vi "IIR_test.vi"() -> ()   [LabVIEW 2017]
uses:
  <vilib>/Analysis/4window.llb/windowTd.ctl
  <vilib>/Utility/file.llb/Read Delimited Spreadsheet (DBL).vi
  <vilib>/Analysis/3filter.llb/IIR Filter (DBL).vi
  <vilib>/measure/maspectr.llb/FFT Spectrum (Mag-Phase) for 1 Chan.vi
  <vilib>/measure/NI_MAPro.lvlib
  <vilib>/Analysis/NI_AALPro.lvlib
  <vilib>/Analysis/NI_AALBase.lvlib
  <vilib>/measure/NI_MABase.lvlib
panel:
  out "Phase 3":cluster{"f0":dbl, "df":dbl, "magnitude":dbl[]}(graph)
  out "Magnitude 3":cluster{"f0":dbl, "df":dbl, "magnitude":dbl[]}(graph)
  out "Waveform Graph 3":waveform(dbl)(graph)
  out "error":i32
  out "Phase 2":cluster{"f0":dbl, "df":dbl, "magnitude":dbl[]}(graph)
  out "Magnitude 2":cluster{"f0":dbl, "df":dbl, "magnitude":dbl[]}(graph)
  out "Waveform Graph 2":waveform(dbl)(graph)
  out "Phase":cluster{"f0":dbl, "df":dbl, "magnitude":dbl[]}(graph)
  out "Magnitude":cluster{"f0":dbl, "df":dbl, "magnitude":dbl[]}(graph)
  out "Waveform Graph":waveform(dbl)(graph)
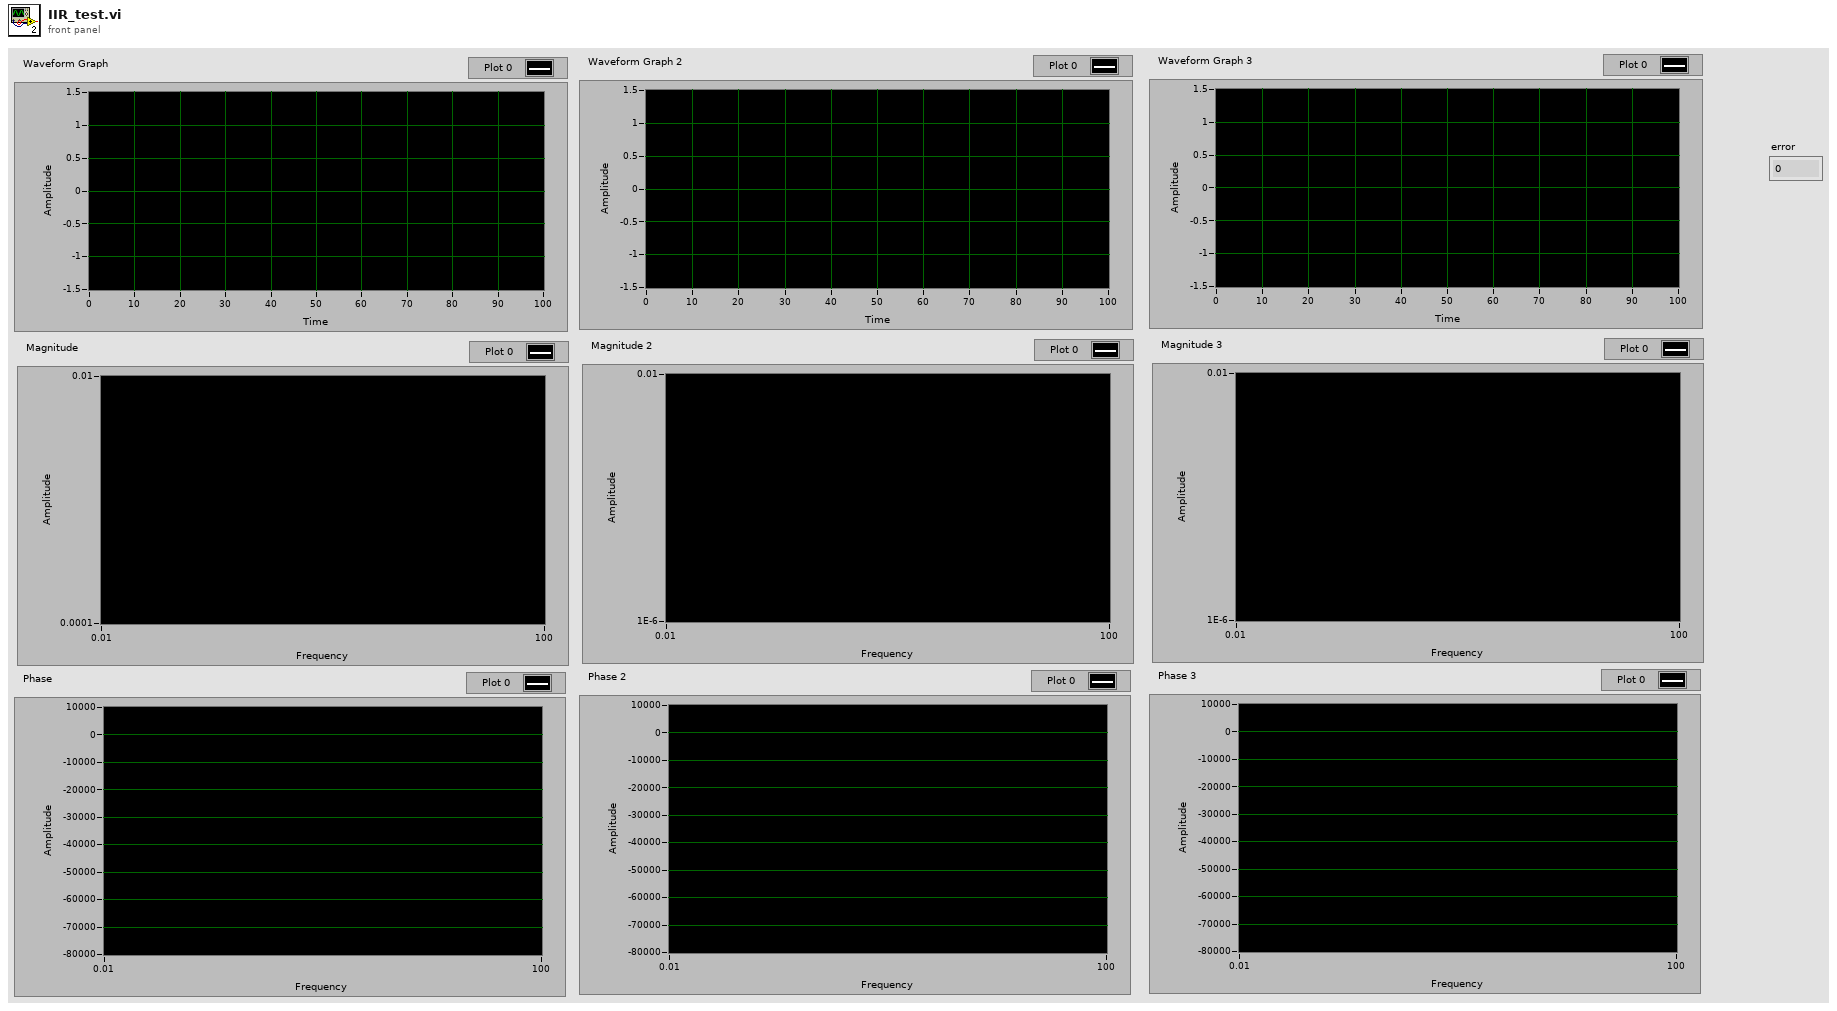
[diagram p1: front panel]
types:
  T1 = typedef "NI_AALPro.lvlib/windowTd.ctl" = u32
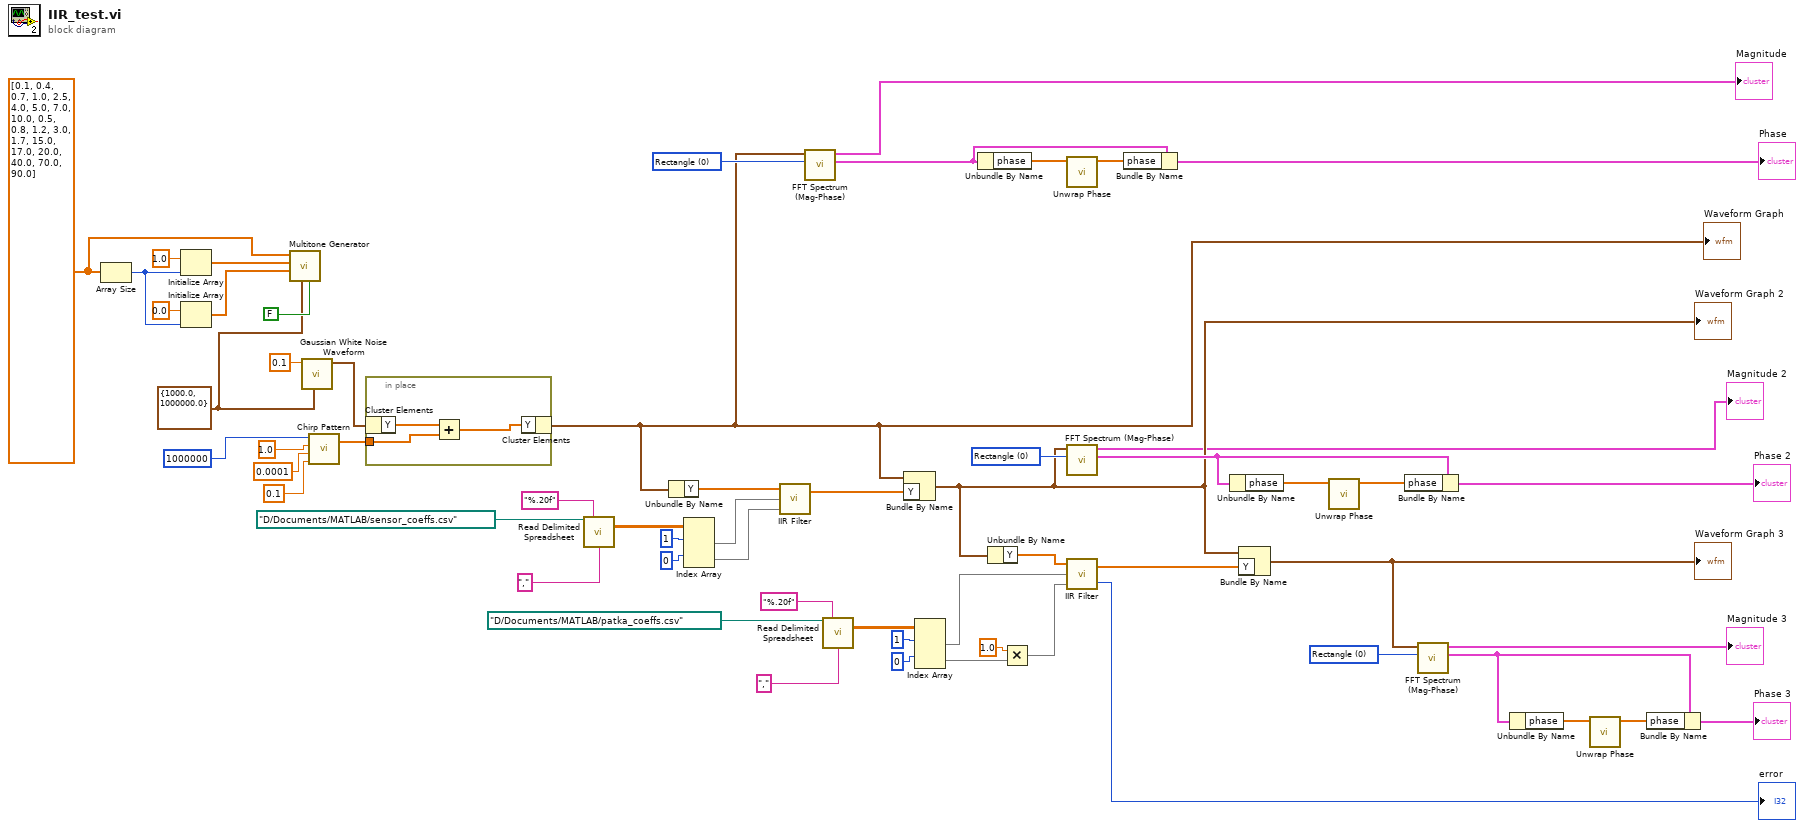
[diagram p0: block diagram]
diagram:
  w25 = T1 0 items=["Rectangle"=0, "Hanning"=1, "Hamming"=2, "Blackman-Harris"=3, "Exact Blackman"=4, "Blackman"=5, "Flat Top"=6, "4 Term B-Harris "=7, "7 Term B-Harris"=8, "Low Sidelobe"=9, "Blackman Nuttall"=11, "Triangle"=30, "Bartlett-Hanning"=31, "Bohman"=32, "Parzen"=33, "Welch"=34, "Kaiser"=60, "Dolph-Chebyshev"=61, "Gaussian"=62] ("window")
  w51 = T1 0 items=["Rectangle"=0, "Hanning"=1, "Hamming"=2, "Blackman-Harris"=3, "Exact Blackman"=4, "Blackman"=5, "Flat Top"=6, "4 Term B-Harris "=7, "7 Term B-Harris"=8, "Low Sidelobe"=9, "Blackman Nuttall"=11, "Triangle"=30, "Bartlett-Hanning"=31, "Bohman"=32, "Parzen"=33, "Welch"=34, "Kaiser"=60, "Dolph-Chebyshev"=61, "Gaussian"=62] ("window")
  w58 = T1 0 items=["Rectangle"=0, "Hanning"=1, "Hamming"=2, "Blackman-Harris"=3, "Exact Blackman"=4, "Blackman"=5, "Flat Top"=6, "4 Term B-Harris "=7, "7 Term B-Harris"=8, "Low Sidelobe"=9, "Blackman Nuttall"=11, "Triangle"=30, "Bartlett-Hanning"=31, "Bohman"=32, "Parzen"=33, "Welch"=34, "Kaiser"=60, "Dolph-Chebyshev"=61, "Gaussian"=62] ("window")
  w55 = dbl[] [0.1, 0.4, 0.7, 1.0, 2.5, 4.0, 5.0, 7.0, 10.0, 0.5, 0.8, 1.2, 3.0, 1.7, 15.0, 17.0, 20.0, 40.0, 70.0, 90.0]
  w7 = cluster{"Fs":dbl, "#s":dbl} {"Fs"=1000.0, "#s"=1000000.0} ("sampling info")
  n1 = Array Size(array=w55) -> (size(s)=w54:i32)
  n2 = Initialize Array(1.0 ("element"), w54) -> (w56:dbl[])
  n3 = Initialize Array(0.0 ("element"), w54) -> (w57:dbl[])
  n4 = call <vilib>:"Multitone Generator.vi"("coerce frequencies?"=FALSE, "sampling info"=w7, "tone phases"=w57, "tone amplitudes"=w56, "tone frequencies"=w55) -> ()  [unwired: 3 in, 4 out]
  n5 = call <vilib>:"Gaussian White Noise Waveform.vi"("sampling info"=w7, "standard deviation"=0.1) -> ("signal out"=w8:waveform(dbl))  [unwired: 8 in, 1 out]
  n6 = call <vilib>:"Chirp Pattern.vi"("f2"=0.1, "f1"=0.0001, "amplitude"=1.0, "samples"=1000000) -> ("Chirp Pattern"=w2:dbl[])  [unwired: 1 out]
  n7 = in-place {
    in-place-border: w2 -> [w60]
    n8 = in-place-cluster #1(w8) -> ("Y"=w62:dbl[])
    n9 = Add(x=w62, y=w60) -> (x+y=w61:dbl[])
    n10 = in-place-cluster #1("Y"=w61) -> (w1:waveform(dbl))
  }
  "Waveform Graph" <- w1
  n11 = call-poly <vilib>:"Read Delimited Spreadsheet.vi"("file path (dialog if empty)"=path "D:/Documents/MATLAB/sensor_coeffs.csv", "format (%.3f)"="%.20f", "delimiter (\\t)"="," ("delimiter (\\t)")) -> ("all rows"=w27:dbl[][])  [unwired: 7 in, 5 out]
  n12 = Unbundle By Name(w1) -> ("Y"=w28:dbl[])
  n13 = Index Array(array=w27, index (row) #1=1 ("index (row)"), index (row) #2=0 ("index (row)")) -> (element #1=w29:dbl[], element #2=w30:dbl[])  [unwired: 2 in]
  n14 = call-poly <vilib>:"IIR Filter.vi"("Forward Coefficients"=w30, "Reverse Coefficients"=w29, "X"=w28) -> ("Filtered X"=w26:dbl[])  [unwired: 1 in, 1 out]
  n15 = call-poly <vilib>:"FFT Spectrum (Mag-Phase).vi"("window"=w25, "time signal"=w1) -> ("phase"=w22:cluster{"f0":dbl, "df":dbl, "phase":dbl[]}, "magnitude"=→"Magnitude":cluster{"f0":dbl, "df":dbl, "magnitude":dbl[]})  [unwired: 5 in, 3 out]
  n16 = call-poly <vilib>:"Read Delimited Spreadsheet.vi"("file path (dialog if empty)"=path "D:/Documents/MATLAB/patka_coeffs.csv", "format (%.3f)"="%.20f", "delimiter (\\t)"="," ("delimiter (\\t)")) -> ("all rows"=w49:dbl[][])  [unwired: 7 in, 5 out]
  n17 = Bundle By Name(cluster=w1, "Y"=w26) -> (w16:waveform(dbl))
  "Waveform Graph 2" <- w16
  n18 = Index Array(array=w49, index (row) #1=1 ("index (row)"), index (row) #2=0 ("index (row)")) -> (element #1=w11:dbl[], element #2=w10:dbl[])  [unwired: 2 in]
  n19 = Unbundle By Name(w22) -> ("phase"=w24:dbl[])
  n20 = Unbundle By Name(w16) -> ("Y"=w46:dbl[])
  n21 = Multiply(x=1.0, y=w10) -> (x*y=w12:dbl[])
  n22 = call <vilib>:"Unwrap Phase.vi"("Phase"=w24) -> ("Unwrapped Phase"=w23:dbl[])  [unwired: 9 in, 1 out]
  n23 = call-poly <vilib>:"FFT Spectrum (Mag-Phase).vi"("window"=w58, "time signal"=w16) -> ("phase"=w41:cluster{"f0":dbl, "df":dbl, "phase":dbl[]}, "magnitude"=→"Magnitude 2":cluster{"f0":dbl, "df":dbl, "magnitude":dbl[]})  [unwired: 5 in, 3 out]
  n24 = call-poly <vilib>:"IIR Filter.vi"("Forward Coefficients"=w12, "Reverse Coefficients"=w11, "X"=w46) -> ("error"=→"error":i32, "Filtered X"=w45:dbl[])  [unwired: 1 in]
  n25 = Bundle By Name(cluster=w22, "phase"=w23) -> (→"Phase":cluster{"f0":dbl, "df":dbl, "phase":dbl[]})
  n26 = Unbundle By Name(w41) -> ("phase"=w43:dbl[])
  n27 = Bundle By Name(cluster=w16, "Y"=w45) -> (w17:waveform(dbl))
  "Waveform Graph 3" <- w17
  n28 = call <vilib>:"Unwrap Phase.vi"("Phase"=w43) -> ("Unwrapped Phase"=w42:dbl[])  [unwired: 9 in, 1 out]
  n29 = Bundle By Name(cluster=w41, "phase"=w42) -> (→"Phase 2":cluster{"f0":dbl, "df":dbl, "phase":dbl[]})
  n30 = call-poly <vilib>:"FFT Spectrum (Mag-Phase).vi"("window"=w51, "time signal"=w17) -> ("phase"=w38:cluster{"f0":dbl, "df":dbl, "phase":dbl[]}, "magnitude"=→"Magnitude 3":cluster{"f0":dbl, "df":dbl, "magnitude":dbl[]})  [unwired: 5 in, 3 out]
  n31 = Unbundle By Name(w38) -> ("phase"=w40:dbl[])
  n32 = call <vilib>:"Unwrap Phase.vi"("Phase"=w40) -> ("Unwrapped Phase"=w39:dbl[])  [unwired: 9 in, 1 out]
  n33 = Bundle By Name(cluster=w38, "phase"=w39) -> (→"Phase 3":cluster{"f0":dbl, "df":dbl, "phase":dbl[]})
